vi "test_Study Imponator.vi"() -> ()   [LabVIEW 2023]
uses:
  Study/Study Actor/Study Actor/Study Actor.lvclass
  C:/Program Files/National Instruments/LabVIEW 2023/vi.lib/MGI/Panel Manager/Panel Actor/Panel Actor/Panel Actor.lvclass
  <vilib>/ni/Actors/Network Endpoint Actors/Protocols/Network Stream Strategy/Network Stream/Network Stream.lvclass/Network Stream.ctl
  <vilib>/ni/Actors/Network Endpoint Actors/Protocols/Network Stream Strategy/Network Stream Initiator/Network Stream Initiator.lvclass/Network Stream Initiator.ctl
  Study/Study Actor/Study Actor/Study Actor.lvclass/Study Actor.ctl
  <vilib>/MGI/Panel Manager/Panel/Window Position/Maximize/Maximize.vi
  <vilib>/ni/Actors/Network Endpoint Actors/Protocols/Network Stream Strategy/Network Stream/Write Buffer Size.vi
  <vilib>/ni/Actors/Network Endpoint Actors/Protocols/Network Stream Strategy/Network Stream/Write Name.vi
  <vilib>/MGI/Panel Manager/Panel/Window Position/Maximize/Maximize.lvclass
  C:/Program Files/National Instruments/LabVIEW 2023/vi.lib/MGI/Panel Manager/Panel/Window Position/Window Position.lvclass
  <vilib>/ni/Actors/Network Endpoint Actors/Protocols/Network Stream Strategy/Network Stream Initiator/Network Stream Initiator.lvclass
  C:/Program Files/National Instruments/LabVIEW 2023/vi.lib/ni/Actors/Network Endpoint Actors/Protocols/Network Stream Strategy/Network Stream/Network Stream.lvclass
  C:/Program Files/National Instruments/LabVIEW 2023/vi.lib/ni/Actors/Network Endpoint Actors/Abstract Classes/Message Stream/Message Stream.lvclass
  <vilib>/ni/Actors/Network Endpoint Actors/Protocols/Network Stream Strategy/Network Stream/Write Address.vi
  <vilib>/MGI/Panel Manager/Panel Actor/Panel Actor/Launch Root Panel Window.vi
  <vilib>/MGI/Panel Manager/Panel Actor/Panel Actor/Panel Actor.lvclass
  <vilib>/MGI/Panel Manager/Panel/Panel.lvlib
  C:/Program Files/National Instruments/LabVIEW 2023/vi.lib/MGI/Panel Manager/Panel/Window Position/Maximize/Maximize.lvclass
  C:/Program Files/National Instruments/LabVIEW 2023/vi.lib/ActorFramework/Actor/Actor.lvclass
  D:/git/HAL/HAL GOOP4/Study/Study Actor/Study Actor/Study Actor.lvclass
  D:/git/HAL/HAL GOOP4/Study/Study Actor/IStudy Actor/IStudy Actor.lvclass
  C:/Program Files/National Instruments/LabVIEW 2023/vi.lib/ni/Actors/Network Endpoint Actors/Nested Endpoint Caller/Nested Endpoint Caller/Nested Endpoint Caller.lvclass
panel:
  out "Error Out":errorcluster
  # "HOST"
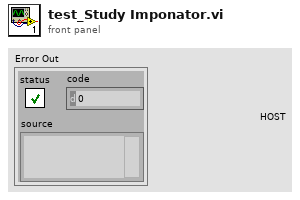
[diagram p1: front panel]
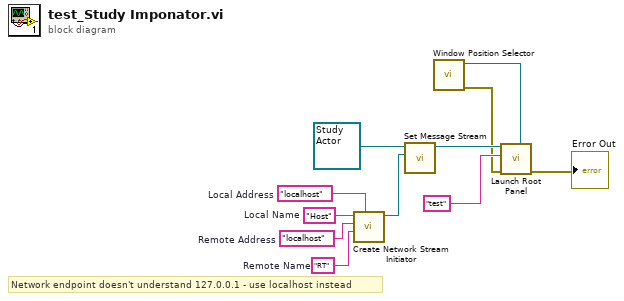
[diagram p0: block diagram]
diagram:
  w5 = "RT"  # Remote Name
  w4 = "localhost"  # Local Address
  w6 = "localhost"  # Remote Address
  w7 = "Host"  # Local Name
  # "Network endpoint doesn't understand 127.0.0.1 - use localhost instead"
  n1 = call <vilib>:"Create Network Stream Initiator.vi"("Local Address"=w4, "Remote Name"=w5, "Remote Address"=w6, "Name"=w7) -> ("Network Stream Initiator out"=w3:refnum<class "Network Stream Initiator.lvclass">)  [unwired: 7 in]
  n2 = call "Set Message Stream.vi"("Message Stream.lvclass"=w3, "Study Actor in"=refnum<class "Study Actor.lvclass"> refnum ("HAL GOOP4.lvlib:Study Actor.lvlib:Study Actor.lvclass")) -> ("Study Actor out"=w8:refnum<class "Study Actor.lvclass">)  [unwired: 9 in]
  n3 = call-poly <vilib>:"Window Position Selector.vi"() -> ("Error Out"=w2:errorcluster, "Maximize out"=w10:refnum<class "Maximize.lvclass">)  [unwired: 10 in]
  n4 = call-poly <vilib>:"Launch Root Panel.vi"("Window Position (Maximize First Call)"=w10, "Error In"=w2, "Title"="test", "Panel Actor in"=w8) -> ("Error Out"=→"Error Out":errorcluster)  [unwired: 6 in, 1 out]
